vi "zgeru - General Matrix Rank-1 Update (CDB).vi"(6 "alpha":cdb=1.0+0.0i, 9 "A":T1, 10 "y":cdb[](array[numeric]), 11 "x":cdb[](array[numeric])) -> (0 "error":i32, 3 "zgeru":T1)   [LabVIEW 2017, in "NI_AALBLAS.lvlib"]
doc: "Calculates the rank-1 update of a general matrix."
uses:
  NI_AALBLAS.lvlib
  ComplexMatrix.ctl
  Fucntion.ctl
  Order.ctl
  BLAS2 Utility(CDB).vi
  NI_Matrix.lvlib
panel:
  # "zgeru=alpha*x*y'+A"
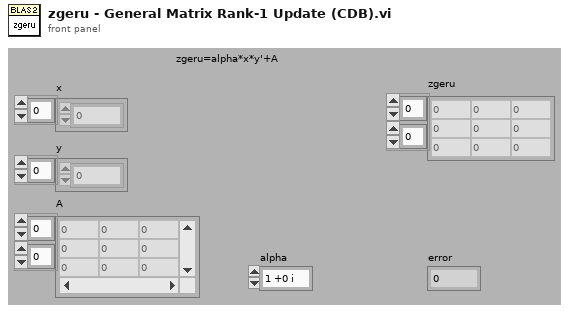
[diagram p1: front panel]
types:
  T1 = typedef "NI_Matrix.lvlib/ComplexMatrix.ctl" = cdb[][]
  T2 = typedef "NI_AALBLAS.lvlib/Order.ctl" = i32
  T3 = typedef "NI_AALBLAS.lvlib/fucntion.ctl" = u16
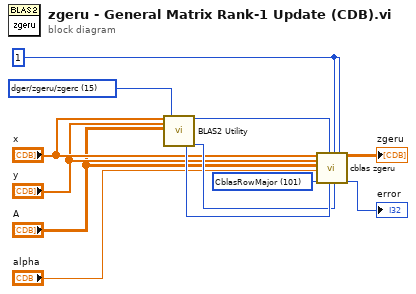
[diagram p0: block diagram]
diagram:
  w1 = T2 101 items=["CblasRowMajor"=101, "CblasColMajor"=102] ("order")
  w2 = 1
  w4 = T3 15 items=["ddot/zdotu/zdotc", "daxpy/zaxpy", "dnrm2/dznrm2", "dasum/dzasum", "dcopy/zcopy", "dswap/zswap", "drotm", "drot/zdrot", "idamax/izamax", "idamin/izamin", "dgemv/zgemv", "dsymv/zhemv", "dtrmv/ztrmv", "dsyr/zher", "dsyr2/zher2", "dger/zgeru/zgerc", "dtrsv/ztrsv", "dgemm/zgemm", "dsymm/zsymm/zhemm", "dtrmm/ztrmm", "dsyrk/zsyrk/zherk", "dsyr2k/zsyr2k/zher2k", "dtrsm/ztrsm"] ("function")
  n1 = call-poly "BLAS2 Utility.vi"("x"="x", "y"="y", "A"="A", "function"=w4) -> ("m"=w12:i32, "lda"=w3:i32, "n"=w11:i32)  [unwired: 1 in, 12 out]
  n2 = call "cblas zgeru.vi"("x"="x", "y"="y", "A"="A", "alpha"="alpha", "order"=w1, "lda"=w3, "m"=w12, "incx"=w2, "n"=w11, "incy"=w2) -> ("zgeru"=→"zgeru":T1, "error"=→"error":i32)  [unwired: 8 out]
